vi "Lift To Inch.vi"(7 "HP Speed":dbl=0.95, 11 "Inches to move":dbl) -> (2 "Done":bool=TRUE)   [LabVIEW 2014]
uses:
  Begin/Global Variables.vi
  <vilib>/Rock Robotics/Network Tables/SD Write Boolean.vi
  Begin/Global RefNums.vi
  <vilib>/Rock Robotics/Network Tables/SD Write Number.vi
panel:
  in  "Down Speed":dbl=0.75
  in  "homing right PID":T1={"proportional gain (Kc)"=0.0007, "integral time (Ti, min)"=0.0, "derivative time (Td, min)"=0.0003} {"derivative time (Td, min)" format="%.4f"; "integral time (Ti, min)" format="%.6f"; "proportional gain (Kc)" format="%.5f"}
  in  "homing left PID":T2={"proportional gain (Kc)"=0.002, "integral time (Ti, min)"=0.0, "derivative time (Td, min)"=0.0005} {"derivative time (Td, min)" format="%.10f"; "proportional gain (Kc)" format="%.5f"}
  in  "Output Range 2":cluster{"output high":dbl, "output low":dbl}={"output high"=0.5, "output low"=-0.5} {"output low" format="%.2f"; "output high" format="%.2f"}
  in  "Increase":dbl=0.3 format="%#_13g"
  in  "lower limit 2":dbl=0.5 format="%#_13g"
  in  "lower limit":dbl=0.5
  in  "normalize":dbl=0.834
  in  "inches slowed":dbl=10.0
  in  "Dec Constant":dbl=-2.0
  in  "LF Speed":dbl=0.6
  in  "slave offset":dbl=1800.0
  in  "Ramp right PID gains":T1={"proportional gain (Kc)"=0.0006, "integral time (Ti, min)"=0.0, "derivative time (Td, min)"=0.0} {"derivative time (Td, min)" format="%.4f"; "integral time (Ti, min)" format="%.6f"; "proportional gain (Kc)" format="%.5f"}
  in  "Ramp left PID gains":T2={"proportional gain (Kc)"=0.0046, "integral time (Ti, min)"=0.005499999970197678, "derivative time (Td, min)"=0.0001} {"derivative time (Td, min)" format="%.10f"; "proportional gain (Kc)" format="%.5f"}
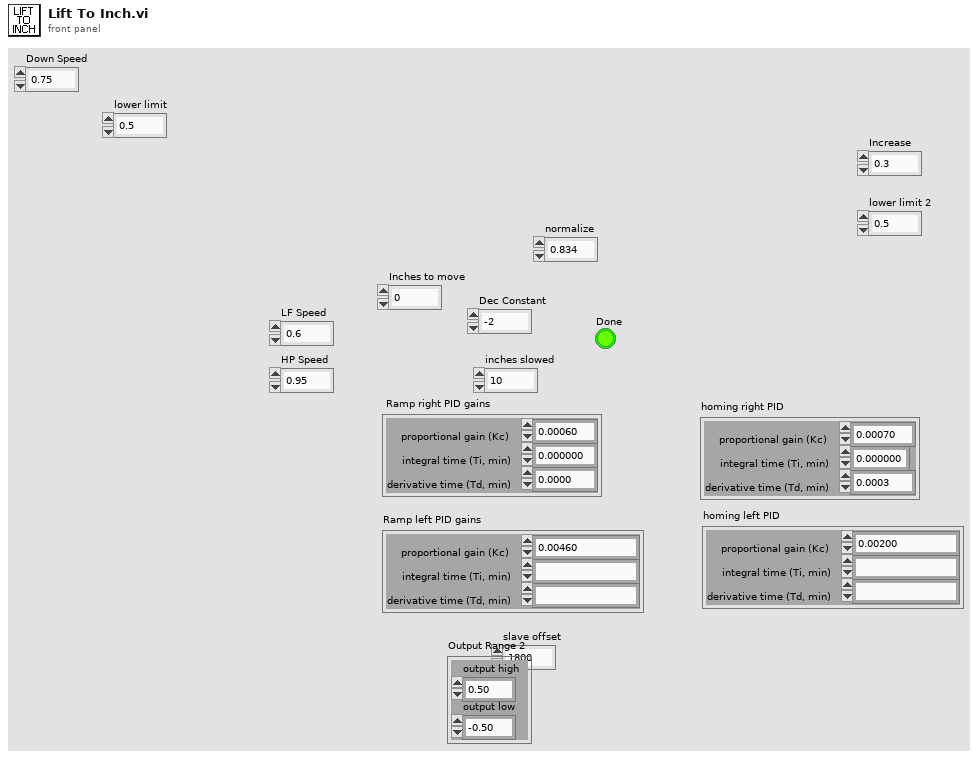
[diagram p1: front panel]
types:
  T1 = cluster{"proportional gain (Kc)":dbl, "integral time (Ti, min)":dbl, "derivative time (Td, min)":dbl}
  T2 = cluster{"proportional gain (Kc)":dbl, "integral time (Ti, min)":fxp<+/-,64,32>, "derivative time (Td, min)":dbl}
  T3 = typedef "WPI_EncoderDevRef.ctl" = cluster{"DevStatus":errorcluster, "EncoderIndex":T4, "CounterIndex":T5, "DistancePerCount":dbl, "Decoding Type":T6}
  T4 = typedef "FPGA_EncoderIdx.ctl" = enum8{"Enc 0", "Enc 1", "Enc 2", "Enc 3", "Enc 4", "Enc 5", "Enc 6", "Enc 7", "Invalid"}
  T5 = typedef "FPGA_CounterCtrSystemIndex.ctl" = enum8{"Ctr 0", "Ctr 1", "Ctr 2", "Ctr 3", "Ctr 4", "Ctr 5", "Ctr 6", "Ctr 7", "Invalid"}
  T6 = typedef "WPI_EncoderType.ctl" = enum16{"1x", "2x", "4x"}
  T7 = typedef "WPI_MotorControlDeviceRef.ctl" = cluster{"DeviceStatus":errorcluster, "Type":T8, "PWM":cluster{"Controller":T9, "PWM Channel":T10, "DeadBand":T11}, "CAN":cluster{"Device Number":u8, "Control Mode":T12, "Semaphore":T13, "Max Vout":dbl, "TalonSRX Control Mode":T14}, "Invert":bool, "TransformRef":T15, "InvTransformRef":T15}
  T8 = typedef "WPI_MotorControlType.ctl" = enum16{"PWM", "CAN", "CANTalonSRX"}
  T9 = typedef "FPGA_TypedefDigitalModule.ctl" = enum16{"Controller 1"}
  T10 = typedef "FPGA_DIOPWMChannel.ctl" = enum8{"PWM 0", "PWM 1", "PWM 2", "PWM 3", "PWM 4", "PWM 5", "PWM 6", "PWM 7", "PWM 8", "PWM 9", "PWM MXP 0", "PWM MXP 1", "PWM MXP 2", "PWM MXP 3", "PWM MXP 4", "PWM MXP 5", "PWM MXP 6", "PWM MXP 7", "PWM MXP 8", "PWM MXP 9", "Invalid"}
  T11 = typedef "WPI_PWMDeadband.ctl" = cluster{"Name":string, "maxPositivePwm":i32, "minPositivePwm":i32, "centerPwm":i32, "maxNegativePwm":i32, "minNegativePwm":i32, "angularRange":u16}
  T12 = typedef "WPI_CANJaguar_ControlMode.ctl" = enum8{"Percent VBus", "Current", "Speed", "Position", "Voltage"}
  T13 = typedef "Semaphore RefNum" = refnum<k1>
  T14 = typedef "WPI_CANTalonSRX_APIControlMode.ctl" = enum8{"Percent VBus", "Speed", "Position", "Slave", "Unchanged / Invalid"}
  T15 = typedef "WPI_PWMTransform_ConPane.ctl" = refnum<vi>
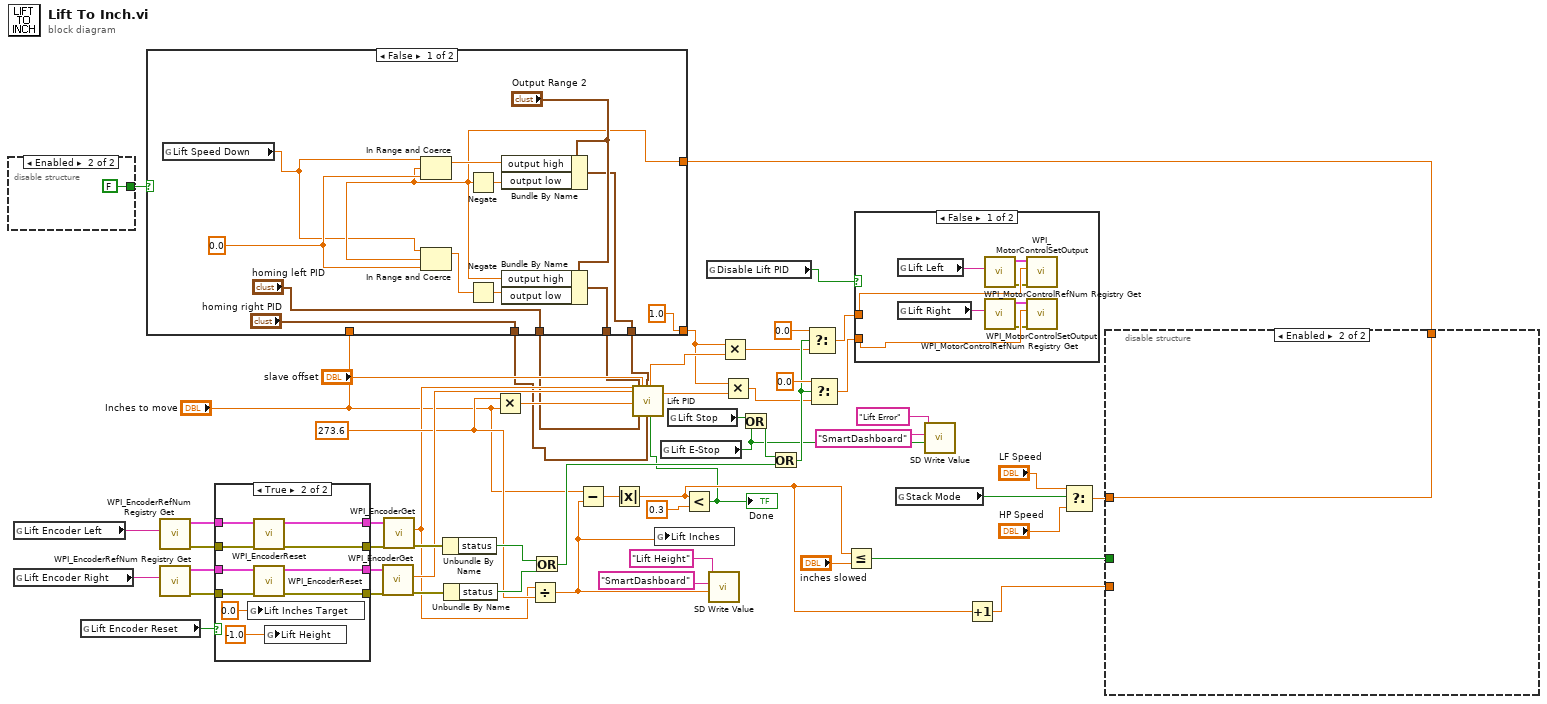
[diagram p0: block diagram]
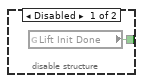
[diagram p2: hidden frame]
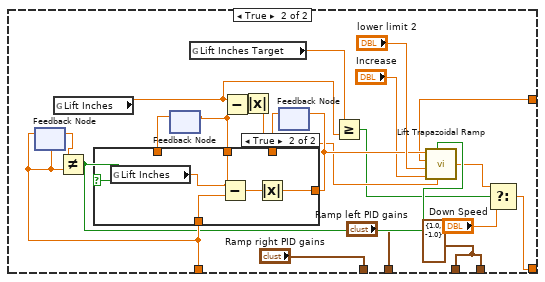
[diagram p3: hidden frame]
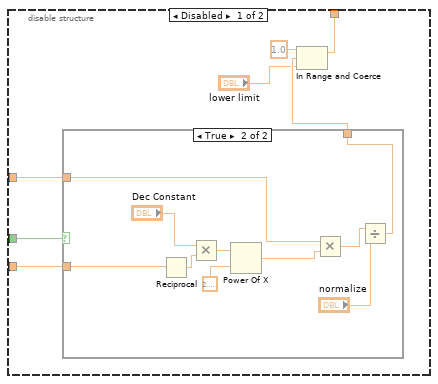
[diagram p6: hidden frame]
diagram:
  w25 = 273.6 ("y")
  n1 = disable-structure shown="Enabled" {
    disable-tunnel: [w59 FALSE ("Lift Init Done")] -> w10
    frame Disabled {
      n2 = global read "Global Variables.vi" "Lift Init Done"() -> (w59:bool)
    }
    frame Enabled {
    }
  }
  n3 = global read "Global RefNums.vi" "Lift Encoder Left"() -> (w35:string)
  n4 = global read "Global RefNums.vi" "Lift Encoder Right"() -> (w34:string)
  n5 = global read "Global Variables.vi" "Lift Encoder Reset"() -> (w24:bool)
  n6 = call <vilib>:"WPI_EncoderRefNum Registry Get.vi"("refnum name"=w35) -> ("error out"=w53:errorcluster, "EncoderDevRef"=w52:T3)  [unwired: 9 in]
  n7 = call <vilib>:"WPI_EncoderRefNum Registry Get.vi"("refnum name"=w34) -> ("error out"=w50:errorcluster, "EncoderDevRef"=w51:T3)  [unwired: 9 in]
  n8 = case shown="True" w24 {
    tunnel: w50 -> [w61 w74]
    tunnel: w51 -> [w62 w73]
    tunnel: w53 -> [w63 w71]
    tunnel: w52 -> [w64 w72]
    tunnel: [w64 w70] -> w55
    tunnel: [w62 w69] -> w56
    tunnel: [w61 w68] -> w57
    tunnel: [w63 w67] -> w58
    frame False {
    }
    frame True {
      n9 = global write "Global Variables.vi" "Lift Inches Target"(0.0 ("Lift Inches Target")) -> ()
      n10 = call <vilib>:"WPI_EncoderReset.vi"("error in (no error)"=w71, "EncoderDevRef"=w72) -> ("error out"=w67:errorcluster, "EncoderDevRef"=w70:T3)  [unwired: 8 in]
      n11 = call <vilib>:"WPI_EncoderReset.vi"("error in (no error)"=w74, "EncoderDevRef"=w73) -> ("error out"=w68:errorcluster, "EncoderDevRef"=w69:T3)  [unwired: 8 in]
      n12 = global write "Global Variables.vi" "Lift Height"(-1.0 ("Lift Inches Target")) -> ()
    }
  }
  n13 = call <vilib>:"WPI_EncoderGet.vi"("error in (no error)"=w57, "EncoderDevRef"=w56) -> ("error out"=w39:errorcluster, "Distance"=w32:dbl)  [unwired: 4 in, 4 out]
  n14 = call <vilib>:"WPI_EncoderGet.vi"("error in (no error)"=w58, "EncoderDevRef"=w55) -> ("error out"=w42:errorcluster, "Distance"=w23:dbl)  [unwired: 4 in, 4 out]
  n15 = Unbundle By Name(w42) -> ("status"=w40:bool)
  n16 = Unbundle By Name(w39) -> ("status"=w38:bool)
  n17 = Multiply(x=w25, y="Inches to move") -> (x*y=w49:dbl)
  n18 = Divide(x=w23, y=w25) -> (x/y=w29:dbl)
  n19 = Or(x=w40, y=w38) -> (x .or. y?=w37:bool)
  n20 = Subtract(x="Inches to move", y=w29) -> (x-y=w48:dbl)
  n21 = Absolute Value(x=w48) -> (abs(x)=w21:dbl)
  n22 = global write "Global Variables.vi" "Lift Inches"(w29) -> ()
  n23 = global read "Global Variables.vi" "Lift E-Stop"() -> (w26:bool)
  n24 = global read "Global Variables.vi" "Lift Stop"() -> (w33:bool)
  n25 = Less?(x=w21, y=0.3) -> (x < y?=w5:bool)
  "Done" <- w5
  n26 = global read "Global Variables.vi" "Disable Lift PID"() -> (w17:bool)
  n27 = call-poly <vilib>:"SD Write Value.vi"("Numeric"=w29, "Table Prefix"="SmartDashboard", "Name"="Lift Height") -> ()  [unwired: 7 in, 2 out]
  n28 = Or(x=w33, y=w26) -> (x .or. y?=w36:bool)
  n29 = Or(x=w36, y=w37) -> (x .or. y?=w41:bool)
  n30 = Less Or Equal?(x=w21, y="inches slowed") -> (x <= y?=w22:bool)
  n31 = global read "Global Variables.vi" "Stack Mode"() -> (w1:bool)
  n32 = call-poly <vilib>:"SD Write Value.vi"("Boolean"=w26, "Table Prefix"="SmartDashboard", "Name"="Lift Error") -> ()  [unwired: 7 in, 2 out]
  n33 = Increment(x=w21) -> (x+1=w20:dbl)
  n34 = Select(t="LF Speed", s=w1, f="HP Speed") -> (s? t:f=w4:dbl)
  n35 = disable-structure shown="Enabled" {
    disable-tunnel: w22 -> [w81 _]
    disable-tunnel: w4 -> [w80 w93]
    disable-tunnel: w20 -> [w79 _]
    disable-tunnel: [w75 w93] -> w18
    frame Disabled {
      n36 = case shown="True" w81 {
        tunnel: w80 -> [w82 w89]
        tunnel: [w82 w84] -> w78
        tunnel: w79 -> [_ w87]
        frame False {
        }
        frame True {
          n37 = Reciprocal(x=w87) -> (1/x=w86:dbl)
          n38 = Multiply(x="Dec Constant", y=w86) -> (x*y=w90:dbl)
          n39 = Power Of X(1:2.718281828459045, 2:w90) -> (0:w88:dbl)
          n40 = Multiply(x=w89, y=w88) -> (x*y=w85:dbl)
          n41 = Divide(x=w85, y="normalize") -> (x/y=w84:dbl)
        }
      }
      n42 = In Range and Coerce(upper limit=1.0, x=w78, lower limit="lower limit") -> (coerced(x)=w75:dbl)  [unwired: 1 out]
    }
    frame Enabled {
    }
  }
  n43 = case shown="False" w10 {
    tunnel: w18 -> [w98 w111]
    tunnel: [w100 w116] -> w8
    tunnel: "Inches to move" -> [_ w127]
    tunnel: [1.0 ("Speed") w107] -> w13
    tunnel: [w97 w116] -> w9
    tunnel: ["homing left PID" "Ramp left PID gains"] -> w7
    tunnel: ["homing right PID" "Ramp right PID gains"] -> w6
    frame False {
      w104 = 0.0 ("lower limit")
      n44 = global read "Global Variables.vi" "Lift Speed Down"() -> (w94:dbl)
      n45 = In Range and Coerce(upper limit=w94, x=w98, lower limit=w104) -> (coerced(x)=w101:dbl)  [unwired: 1 out]
      n46 = In Range and Coerce(upper limit=w94, x=w98, lower limit=w104) -> (coerced(x)=w105:dbl)  [unwired: 1 out]
      n47 = Negate(x=w98) -> (-x=w102:dbl)
      n48 = Negate(x=w105) -> (-x=w106:dbl)
      n49 = Bundle By Name(cluster="Output Range 2", "output high"=w101, "output low"=w102) -> (w100:cluster{"output high":dbl, "output low":dbl})
      n50 = Bundle By Name(cluster="Output Range 2", "output high"=w98, "output low"=w106) -> (w97:cluster{"output high":dbl, "output low":dbl})
    }
    frame True {
      w116 = cluster{"output high":dbl, "output low":dbl} {"output high"=1.0, "output low"=-1.0} ("left output range")
      n51 = feedback #1(w127) -> (w123:dbl)
      n52 = feedback-in #1(w127) -> ()
      n53 = global read "Global Variables.vi" "Lift Inches"() -> (w113:dbl)
      n54 = Not Equal?(x=w123, y=w127) -> (x != y?=w117:bool)
      n55 = feedback #2() -> (w121:dbl)  [unwired: 1 in]
      n56 = global read "Global Variables.vi" "Lift Inches Target"() -> (w112:dbl)
      n57 = feedback #3() -> (w124:dbl)  [unwired: 1 in]
      n58 = case shown="True" w117 {
        tunnel: w127 -> [_ w132]
        tunnel: [w129 w131] -> w125
        tunnel: w124 -> [w129 _]
        tunnel: [w128 w130] -> w122
        tunnel: w121 -> [w128 _]
        frame False {
        }
        frame True {
          n59 = global read "Global Variables.vi" "Lift Inches"() -> (w130:dbl)
          n60 = Subtract(x=w130, y=w132) -> (x-y=w133:dbl)
          n61 = Absolute Value(x=w133) -> (abs(x)=w131:dbl)
        }
      }
      n62 = feedback-in #2(w122) -> ()
      n63 = Subtract(x=w113, y=w122) -> (x-y=w120:dbl)
      n64 = Absolute Value(x=w120) -> (abs(x)=w119:dbl)
      n65 = feedback-in #3(w125) -> ()
      n66 = Greater Or Equal?(x=w112, y=w113) -> (x >= y?=w109:bool)
      n67 = call "Lift Trapazoidal Ramp.vi"("Encoder"=w119, "Reset"=w117, "Increase"="Increase", "lower limit"="lower limit 2", "Speed (-1 to 1)"=w111, "Distance (inches)"=w125) -> ("Speed"=w110:dbl)
      n68 = Select(t=w110, s=w109, f="Down Speed") -> (s? t:f=w107:dbl)
    }
  }
  n69 = call "Lift PID.vi"("left encoder"=w23, "right encoder"=w32, "move to distance"=w49, "left output range"=w9, "left PID gains"=w7, "slave offset"="slave offset", "right output range"=w8, "right PID gains"=w6, "Reinitialize"=w5) -> ("lift motor left"=w15:dbl, "lift motor right"=w14:dbl)  [unwired: 17 in]
  n70 = Multiply(x=w13, y=w15) -> (x*y=w12:dbl)
  n71 = Multiply(x=w13, y=w14) -> (x*y=w11:dbl)
  n72 = Select(t=0.0, s=w41, f=w12) -> (s? t:f=w44:dbl)
  n73 = Select(t=0.0, s=w41, f=w11) -> (s? t:f=w43:dbl)
  n74 = case shown="False" w17 {
    tunnel: w44 -> [w141 _]
    tunnel: w43 -> [w140 _]
    frame False {
      n75 = global read "Global RefNums.vi" "Lift Left"() -> (w135:string)
      n76 = global read "Global RefNums.vi" "Lift Right"() -> (w134:string)
      n77 = call <vilib>:"WPI_MotorControlRefNum Registry Get.vi"("refnum name"=w135) -> ("error out"=w139:errorcluster, "MotorControlDevRef"=w138:T7)  [unwired: 9 in]
      n78 = call <vilib>:"WPI_MotorControlRefNum Registry Get.vi"("refnum name"=w134) -> ("error out"=w136:errorcluster, "MotorControlDevRef"=w137:T7)  [unwired: 9 in]
      n79 = call <vilib>:"WPI_MotorControlSetOutput.vi"("error in (no error)"=w139, "Output"=w141, "MotorControlDevRef"=w138) -> ()  [unwired: 6 in, 3 out]
      n80 = call <vilib>:"WPI_MotorControlSetOutput.vi"("error in (no error)"=w136, "Output"=w140, "MotorControlDevRef"=w137) -> ()  [unwired: 6 in, 3 out]
    }
    frame True {
    }
  }
